vi "AppendAvi.vi"(9 "aviFile":T1, 10 "frame_convert":T2, 11 "frame_raw":T2) -> (1 "aviFile out":T1, 2 "frame_convert_out":T2, 3 "frame_raw_out":T2)   [LabVIEW 2019]
uses:
  EmergentCameraC/EmergentCameraC.lvlib
types:
  T1 = cluster{"fileName[0]":i8, "fileName[1]":i8, "fileName[2]":i8, "fileName[3]":i8, "fileName[4]":i8, "fileName[5]":i8, "fileName[6]":i8, "fileName[7]":i8, "fileName[8]":i8, "fileName[9]":i8, "fileName[10]":i8, "fileName[11]":i8, "fileName[12]":i8, "fileName[13]":i8, "fileName[14]":i8, "fileName[15]":i8, "fileName[16]":i8, "fileName[17]":i8, "fileName[18]":i8, "fileName[19]":i8, "fileName[20]":i8, "fileName[21]":i8, "fileName[22]":i8, "fileName[23]":i8, "fileName[24]":i8, "fileName[25]":i8, "fileName[26]":i8, "fileName[27]":i8, "fileName[28]":i8, "fileName[29]":i8, "fileName[30]":i8, "fileName[31]":i8, "fileName[32]":i8, "fileName[33]":i8, "fileName[34]":i8, "fileName[35]":i8, "fileName[36]":i8, "fileName[37]":i8, "fileName[38]":i8, "fileName[39]":i8, "fileName[40]":i8, "fileName[41]":i8, "fileName[42]":i8, "fileName[43]":i8, "fileName[44]":i8, "fileName[45]":i8, "fileName[46]":i8, "fileName[47]":i8, "fileName[48]":i8, "fileName[49]":i8, "fileName[50]":i8, "fileName[51]":i8, "fileName[52]":i8, "fileName[53]":i8, "fileName[54]":i8, "fileName[55]":i8, "fileName[56]":i8, "fileName[57]":i8, "fileName[58]":i8, "fileName[59]":i8, "fileName[60]":i8, "fileName[61]":i8, "fileName[62]":i8, "fileName[63]":i8, "fileName[64]":i8, "fileName[65]":i8, "fileName[66]":i8, "fileName[67]":i8, "fileName[68]":i8, "fileName[69]":i8, "fileName[70]":i8, "fileName[71]":i8, "fileName[72]":i8, "fileName[73]":i8, "fileName[74]":i8, "fileName[75]":i8, "fileName[76]":i8, "fileName[77]":i8, "fileName[78]":i8, "fileName[79]":i8, "fileName[80]":i8, "fileName[81]":i8, "fileName[82]":i8, "fileName[83]":i8, "fileName[84]":i8, "fileName[85]":i8, "fileName[86]":i8, "fileName[87]":i8, "fileName[88]":i8, "fileName[89]":i8, "fileName[90]":i8, "fileName[91]":i8, "fileName[92]":i8, "fileName[93]":i8, "fileName[94]":i8, "fileName[95]":i8, "fileName[96]":i8, "fileName[97]":i8, "fileName[98]":i8, "fileName[99]":i8, "fileName[100]":i8, "fileName[101]":i8, "fileName[102]":i8, "fileName[103]":i8, "fileName[104]":i8, "fileName[105]":i8, "fileName[106]":i8, "fileName[107]":i8, "fileName[108]":i8, "fileName[109]":i8, "fileName[110]":i8, "fileName[111]":i8, "fileName[112]":i8, "fileName[113]":i8, "fileName[114]":i8, "fileName[115]":i8, "fileName[116]":i8, "fileName[117]":i8, "fileName[118]":i8, "fileName[119]":i8, "fileName[120]":i8, "fileName[121]":i8, "fileName[122]":i8, "fileName[123]":i8, "fileName[124]":i8, "fileName[125]":i8, "fileName[126]":i8, "fileName[127]":i8, "fileName[128]":i8, "fileName[129]":i8, "fileName[130]":i8, "fileName[131]":i8, "fileName[132]":i8, "fileName[133]":i8, "fileName[134]":i8, "fileName[135]":i8, "fileName[136]":i8, "fileName[137]":i8, "fileName[138]":i8, "fileName[139]":i8, "fileName[140]":i8, "fileName[141]":i8, "fileName[142]":i8, "fileName[143]":i8, "fileName[144]":i8, "fileName[145]":i8, "fileName[146]":i8, "fileName[147]":i8, "fileName[148]":i8, "fileName[149]":i8, "fileName[150]":i8, "fileName[151]":i8, "fileName[152]":i8, "fileName[153]":i8, "fileName[154]":i8, "fileName[155]":i8, "fileName[156]":i8, "fileName[157]":i8, "fileName[158]":i8, "fileName[159]":i8, "fileName[160]":i8, "fileName[161]":i8, "fileName[162]":i8, "fileName[163]":i8, "fileName[164]":i8, "fileName[165]":i8, "fileName[166]":i8, "fileName[167]":i8, "fileName[168]":i8, "fileName[169]":i8, "fileName[170]":i8, "fileName[171]":i8, "fileName[172]":i8, "fileName[173]":i8, "fileName[174]":i8, "fileName[175]":i8, "fileName[176]":i8, "fileName[177]":i8, "fileName[178]":i8, "fileName[179]":i8, "fileName[180]":i8, "fileName[181]":i8, "fileName[182]":i8, "fileName[183]":i8, "fileName[184]":i8, "fileName[185]":i8, "fileName[186]":i8, "fileName[187]":i8, "fileName[188]":i8, "fileName[189]":i8, "fileName[190]":i8, "fileName[191]":i8, "fileName[192]":i8, "fileName[193]":i8, "fileName[194]":i8, "fileName[195]":i8, "fileName[196]":i8, "fileName[197]":i8, "fileName[198]":i8, "fileName[199]":i8, "fileName[200]":i8, "fileName[201]":i8, "fileName[202]":i8, "fileName[203]":i8, "fileName[204]":i8, "fileName[205]":i8, "fileName[206]":i8, "fileName[207]":i8, "fileName[208]":i8, "fileName[209]":i8, "fileName[210]":i8, "fileName[211]":i8, "fileName[212]":i8, "fileName[213]":i8, "fileName[214]":i8, "fileName[215]":i8, "fileName[216]":i8, "fileName[217]":i8, "fileName[218]":i8, "fileName[219]":i8, "fileName[220]":i8, "fileName[221]":i8, "fileName[222]":i8, "fileName[223]":i8, "fileName[224]":i8, "fileName[225]":i8, "fileName[226]":i8, "fileName[227]":i8, "fileName[228]":i8, "fileName[229]":i8, "fileName[230]":i8, "fileName[231]":i8, "fileName[232]":i8, "fileName[233]":i8, "fileName[234]":i8, "fileName[235]":i8, "fileName[236]":i8, "fileName[237]":i8, "fileName[238]":i8, "fileName[239]":i8, "fileName[240]":i8, "fileName[241]":i8, "fileName[242]":i8, "fileName[243]":i8, "fileName[244]":i8, "fileName[245]":i8, "fileName[246]":i8, "fileName[247]":i8, "fileName[248]":i8, "fileName[249]":i8, "fileName[250]":i8, "fileName[251]":i8, "fileName[252]":i8, "fileName[253]":i8, "fileName[254]":i8, "fileName[255]":i8, "codec":i32, "@dummy control@":i8, "@dummy control@":i8, "@dummy control@":i8, "@dummy control@":i8, "fps":dbl, "width":i32, "height":i32, "isColor":i32, "@dummy control@":i8, "@dummy control@":i8, "@dummy control@":i8, "@dummy control@":i8, "privateData":i64}
  T2 = cluster{"pixel_type":u32, "size_x":u32, "size_y":u32, "stride":i32, "offset_x":u32, "offset_y":u32, "padding_x":u32, "padding_y":u32, "trailer_size_y":u32, "frame_id":u16, "@dummy control@":i8, "@dummy control@":i8, "imagePtr":i64, "bufferSize":u32, "@dummy control@":i8, "@dummy control@":i8, "@dummy control@":i8, "@dummy control@":i8, "timestamp":u64, "nsecs":u64, "convertColor":i32, "convertBitDepth":i32, "privateData[0]":u8, "privateData[1]":u8, "privateData[2]":u8, "privateData[3]":u8, "privateData[4]":u8, "privateData[5]":u8, "privateData[6]":u8, "privateData[7]":u8, "privateData[8]":u8, "privateData[9]":u8, "privateData[10]":u8, "privateData[11]":u8, "privateData[12]":u8, "privateData[13]":u8, "privateData[14]":u8, "privateData[15]":u8, "privateData[16]":u8, "privateData[17]":u8, "privateData[18]":u8, "privateData[19]":u8, "privateData[20]":u8, "privateData[21]":u8, "privateData[22]":u8, "privateData[23]":u8, "privateData[24]":u8, "privateData[25]":u8, "privateData[26]":u8, "privateData[27]":u8, "privateData[28]":u8, "privateData[29]":u8, "privateData[30]":u8, "privateData[31]":u8, "privateData[32]":u8, "privateData[33]":u8, "privateData[34]":u8, "privateData[35]":u8, "privateData[36]":u8, "privateData[37]":u8, "privateData[38]":u8, "privateData[39]":u8, "privateData[40]":u8, "privateData[41]":u8, "privateData[42]":u8, "privateData[43]":u8, "privateData[44]":u8, "privateData[45]":u8, "privateData[46]":u8, "privateData[47]":u8, "privateData[48]":u8, "privateData[49]":u8, "privateData[50]":u8, "privateData[51]":u8, "privateData[52]":u8, "privateData[53]":u8, "privateData[54]":u8, "privateData[55]":u8, "privateData[56]":u8, "privateData[57]":u8, "privateData[58]":u8, "privateData[59]":u8, "privateData[60]":u8, "privateData[61]":u8, "privateData[62]":u8, "privateData[63]":u8, "privateData[64]":u8, "privateData[65]":u8, "privateData[66]":u8, "privateData[67]":u8, "privateData[68]":u8, "privateData[69]":u8, "privateData[70]":u8, "privateData[71]":u8, "privateData[72]":u8, "privateData[73]":u8, "privateData[74]":u8, "privateData[75]":u8, "privateData[76]":u8, "privateData[77]":u8, "privateData[78]":u8, "privateData[79]":u8, "privateData[80]":u8, "privateData[81]":u8, "privateData[82]":u8, "privateData[83]":u8, "privateData[84]":u8, "privateData[85]":u8, "privateData[86]":u8, "privateData[87]":u8, "privateData[88]":u8, "privateData[89]":u8, "privateData[90]":u8, "privateData[91]":u8, "privateData[92]":u8, "privateData[93]":u8, "privateData[94]":u8, "privateData[95]":u8, "privateData[96]":u8, "privateData[97]":u8, "privateData[98]":u8, "privateData[99]":u8, "privateData[100]":u8, "privateData[101]":u8, "privateData[102]":u8, "privateData[103]":u8, "privateData[104]":u8, "privateData[105]":u8, "privateData[106]":u8, "privateData[107]":u8, "privateData[108]":u8, "privateData[109]":u8, "privateData[110]":u8, "privateData[111]":u8, "privateData[112]":u8, "privateData[113]":u8, "privateData[114]":u8, "privateData[115]":u8, "privateData[116]":u8, "privateData[117]":u8, "privateData[118]":u8, "privateData[119]":u8, "privateData[120]":u8, "privateData[121]":u8, "privateData[122]":u8, "privateData[123]":u8, "privateData[124]":u8, "privateData[125]":u8, "privateData[126]":u8, "privateData[127]":u8, "privateData[128]":u8, "privateData[129]":u8, "privateData[130]":u8, "privateData[131]":u8, "privateData[132]":u8, "privateData[133]":u8, "privateData[134]":u8, "privateData[135]":u8, "privateData[136]":u8, "privateData[137]":u8, "privateData[138]":u8, "privateData[139]":u8, "privateData[140]":u8, "privateData[141]":u8, "privateData[142]":u8, "privateData[143]":u8, "privateData[144]":u8, "privateData[145]":u8, "privateData[146]":u8, "privateData[147]":u8, "privateData[148]":u8, "privateData[149]":u8, "privateData[150]":u8, "privateData[151]":u8, "privateData[152]":u8, "privateData[153]":u8, "privateData[154]":u8, "privateData[155]":u8, "privateData[156]":u8, "privateData[157]":u8, "privateData[158]":u8, "privateData[159]":u8, "privateData[160]":u8, "privateData[161]":u8, "privateData[162]":u8, "privateData[163]":u8, "privateData[164]":u8, "privateData[165]":u8, "privateData[166]":u8, "privateData[167]":u8, "privateData[168]":u8, "privateData[169]":u8, "privateData[170]":u8, "privateData[171]":u8, "privateData[172]":u8, "privateData[173]":u8, "privateData[174]":u8, "privateData[175]":u8, "privateData[176]":u8, "privateData[177]":u8, "privateData[178]":u8, "privateData[179]":u8, "privateData[180]":u8, "privateData[181]":u8, "privateData[182]":u8, "privateData[183]":u8, "privateData[184]":u8, "privateData[185]":u8, "privateData[186]":u8, "privateData[187]":u8, "privateData[188]":u8, "privateData[189]":u8, "privateData[190]":u8, "privateData[191]":u8, "privateData[192]":u8, "privateData[193]":u8, "privateData[194]":u8, "privateData[195]":u8, "privateData[196]":u8, "privateData[197]":u8, "privateData[198]":u8, "privateData[199]":u8, "privateData[200]":u8, "privateData[201]":u8, "privateData[202]":u8, "privateData[203]":u8, "privateData[204]":u8, "privateData[205]":u8, "privateData[206]":u8, "privateData[207]":u8, "privateData[208]":u8, "privateData[209]":u8, "privateData[210]":u8, "privateData[211]":u8, "privateData[212]":u8, "privateData[213]":u8, "privateData[214]":u8, "privateData[215]":u8, "privateData[216]":u8, "privateData[217]":u8, "privateData[218]":u8, "privateData[219]":u8, "privateData[220]":u8, "privateData[221]":u8, "privateData[222]":u8, "privateData[223]":u8, "privateData[224]":u8, "privateData[225]":u8, "privateData[226]":u8, "privateData[227]":u8, "privateData[228]":u8, "privateData[229]":u8, "privateData[230]":u8, "privateData[231]":u8, "privateData[232]":u8, "privateData[233]":u8, "privateData[234]":u8, "privateData[235]":u8, "privateData[236]":u8, "privateData[237]":u8, "privateData[238]":u8, "privateData[239]":u8, "privateData[240]":u8, "privateData[241]":u8, "privateData[242]":u8, "privateData[243]":u8, "privateData[244]":u8, "privateData[245]":u8, "privateData[246]":u8, "privateData[247]":u8, "privateData[248]":u8, "privateData[249]":u8, "privateData[250]":u8, "privateData[251]":u8, "privateData[252]":u8, "privateData[253]":u8, "privateData[254]":u8, "privateData[255]":u8}
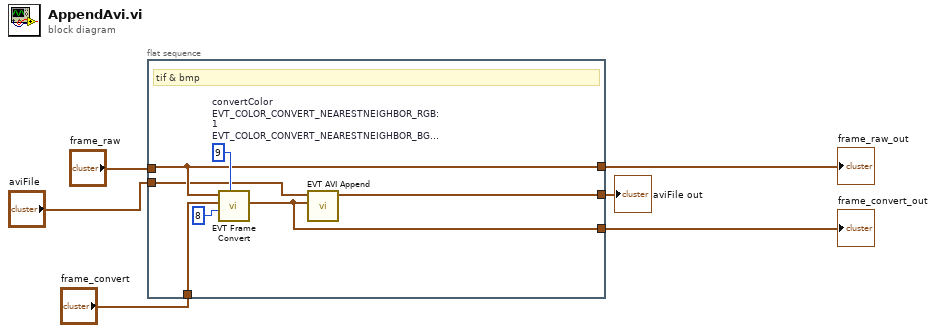
[diagram p0: block diagram]
diagram:
  n1 = flat-sequence {
    tunnel: "frame_convert" -> [w13]
    tunnel: [w7] -> w5
    tunnel: [w10] -> w4
    tunnel: "frame_raw" -> [w10]
    tunnel: "aviFile" -> [w9]
    tunnel: [w8] -> w1
    frame #0 {
      w11 = 9  # convertColor EVT_COLOR_CONVERT_NEARESTNEIGHBOR_RGB: 1 EVT_COLOR_CONVERT_NEARESTNEIGHBOR_BGR: 9
      # "tif & bmp"
      n2 = call "EVT Frame Convert.vi"("convertColor"=w11, "convertBitDepth"=8 ("convertColor"), "frameDst"=w13, "frameSrc"=w10) -> ("frameDst out"=w7:T2)  [unwired: 5 in, 2 out]
      n3 = call "EVT AVI Append.vi"("frame"=w7, "aviFile"=w9) -> ("aviFile out"=w8:T1)  [unwired: 8 in, 1 out]
    }
  }
  "frame_convert_out" <- w5
  "frame_raw_out" <- w4
  "aviFile out" <- w1
